vi "Query - DBL - 2D.vi"(8 "error in":errorcluster, 10 "Query":string, 11 "Module ID":i32=-1) -> (0 "error out":errorcluster, 1 "Meta Data":variant, 2 "Return Data":dbl[][](array[numeric]), 4 "Field Names":string[](array[string]))   [LabVIEW 2014, in "DB_CONNECTOR.lvlib"]
uses:
  DB_CONNECTOR.lvlib
  hse-misc/Conversion/ConvertStringToFloat_Array-2D.vi
  hse-misc/hse-misc.lvlib
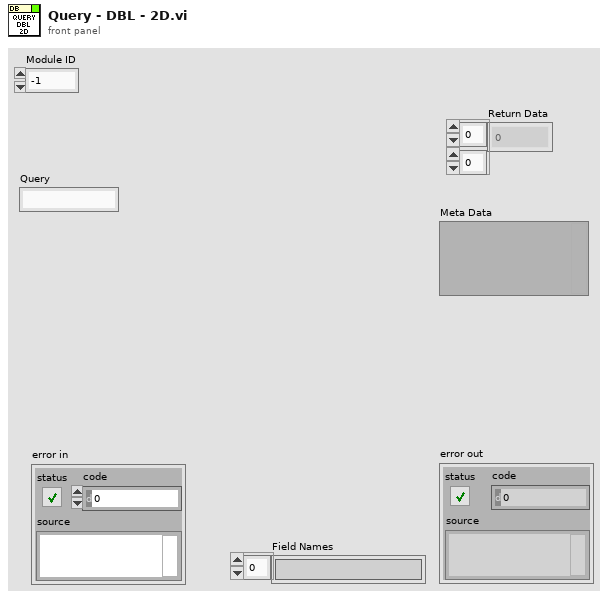
[diagram p1: front panel]
types:
  T1 = typedef "DB_CONNECTOR.lvlib/Query (Reply Payload)--cluster.ctl" = cluster{"Return Data":string[][], "Meta Data":variant, "Field Names":string[], "Query_error":errorcluster}
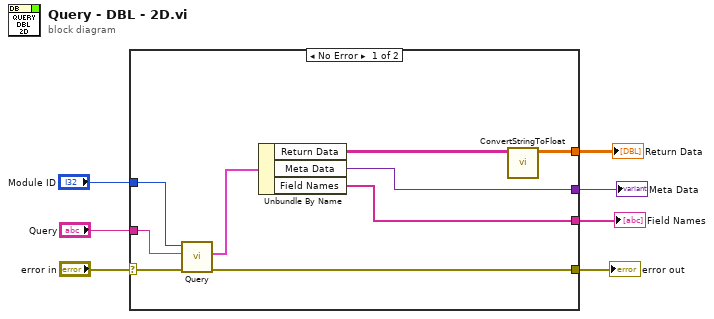
[diagram p0: block diagram]
diagram:
  n1 = case shown="No Error" "error in" {
    selector: "error in" -> [w16 w17]
    tunnel: [w11 w17] -> w6
    tunnel: "Query" -> [w14 _]
    tunnel: "Module ID" -> [w13 _]
    tunnel: [w10 _] -> w2
    tunnel: [w9 _] -> w3
    tunnel: [w8 _] -> w1
    frame No Error {
      n2 = call "Query.vi"("error in (no error)"=w16, "Query"=w14, "Module ID"=w13) -> ("error out"=w11:errorcluster, "Reply Payload"=w15:T1)  [unwired: 7 in]
      n3 = Unbundle By Name(w15) -> ("Return Data"=w12:string[][], "Meta Data"=w10:variant, "Field Names"=w8:string[])
      n4 = call-poly "ConvertStringToFloat.vi"("params"=w12) -> ("Array"=w9:dbl[][])  [unwired: 10 in]
    }
    frame Error {
    }
  }
  "error out" <- w6
  "Return Data" <- w3
  "Meta Data" <- w2
  "Field Names" <- w1
